vi "WPI_SimpleGyro_Get Angle.vi"(8 "error in":errorcluster, 11 "SimpleGyroDevRef":T1 {"Sample Rate" min=0.25 max=100.0 step=0.25}) -> (0 "error out":errorcluster, 1 "Calibrated?":bool, 2 "Angle":dbl, 3 "SimpleGyroDevRef":T1 {"Sample Rate" min=0.25 max=100.0 step=0.25})   [LabVIEW 2016, in "Apple Pi Gyro Library.lvlib" / "SimpleGyro.lvlib"]
doc: "Reads a sample from the SimpleGyro and makes it available to the rest of your program. Use this in your RobotMain.vi to provide WPI_RobotDriveHolonomicDrive.vi angle feedback."
uses:
  SimpleGyro.lvlib
  WPI_SimpleGyroDevRef.ctl
  <vilib>/Rock Robotics/SystemInterfaces/spilib/spi_bus.ctl
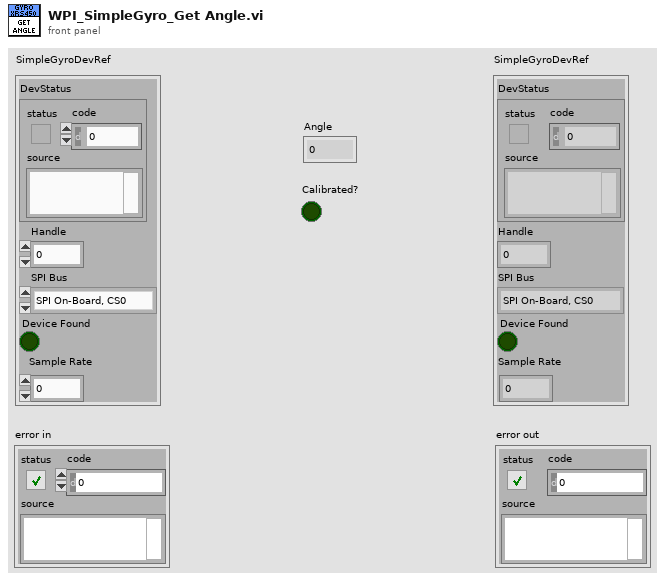
[diagram p1: front panel]
types:
  T1 = typedef "Apple Pi Gyro Library.lvlib/SimpleGyro.lvlib/WPI_SimpleGyroDevRef.ctl" = cluster{"DevStatus":errorcluster, "Handle":i32, "SPI Bus":T2, "Device Found":bool, "Sample Rate":dbl}
  T2 = typedef "spi_bus.ctl" = enum16{"SPI On-Board, CS0", "SPI On-Board, CS1", "SPI On-Board, CS2", "SPI On-Board, CS3", "SPI MXP", "Invalid"}
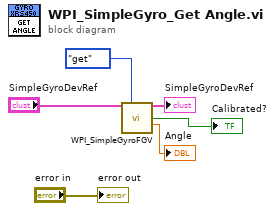
[diagram p0: block diagram]
diagram:
  n1 = call "WPI_SimpleGyroFGV.vi"("SimpleGyroDevRef"="SimpleGyroDevRef", "Operation"=enum16{"set", "get"}."get") -> ("SimpleGyroDevRef"=→"SimpleGyroDevRef":T1, "Calibrated?"=→"Calibrated?":bool, "Angle"=→"Angle":dbl)  [unwired: 9 in, 2 out]
  "error out" <- "error in"
